vi "Delete Profile from File.vi"(8 "error in":errorcluster, 10 "Name":string, 11 "Profile File":path) -> (0 "error out":errorcluster)   [LabVIEW 2025, in "TS Environment Manager.lvlib"]
uses:
  TS Environment Manager.lvlib
  <vilib>/Utility/config.llb/NI_LVConfig.lvlib
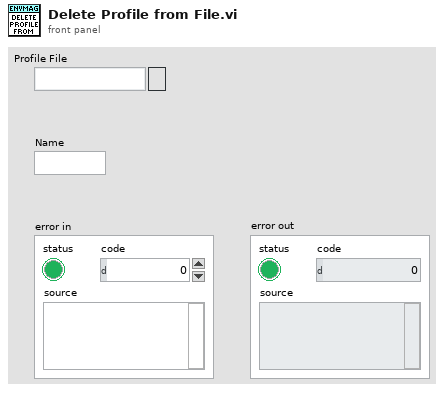
[diagram p1: front panel]
types:
  T1 = typedef "NI_LVConfig.lvlib/Config Data RefNum.ctl" = refnum<k1>
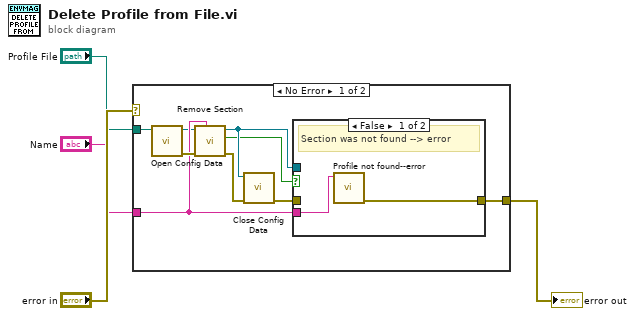
[diagram p0: block diagram]
diagram:
  n1 = case shown="No Error" "error in" {
    selector: "error in" -> [_ w17]
    tunnel: "Name" -> [w8 _]
    tunnel: "Profile File" -> [w5 _]
    tunnel: [w10 w17] -> w3
    frame No Error {
      n2 = call <vilib>:"Open Config Data.vi"("configuration file path"=w5) -> ("error out"=w11:errorcluster, "refnum"=w6:T1)  [unwired: 8 in, 1 out]
      n3 = call <vilib>:"Remove Section.vi"("section"=w8, "error in (no error)"=w11, "refnum"=w6) -> ("error out"=w12:errorcluster, "section exists?"=w7:bool, "refnum out"=w9:T1)  [unwired: 6 in]
      n4 = call <vilib>:"Close Config Data.vi"("error in (no error)"=w12, "refnum"=w9) -> ("error out"=w13:errorcluster)  [unwired: 8 in, 1 out]
      n5 = case shown="False" w7 {
        tunnel: w9 -> [_ _]
        tunnel: w8 -> [w14 _]
        tunnel: w13 -> [_ w16]
        tunnel: [w15 w16] -> w10
        frame False {
          # "Section was not found --> error"
          n6 = call "Profile not found--error.vi"("Name"=w14) -> ("error out"=w15:errorcluster)  [unwired: 10 in]
        }
        frame True {
          # "Section found and deleted"
        }
      }
    }
    frame Error {
      # "Pass error without further action"
    }
  }
  "error out" <- w3
